vi "1.3.5-Confirm.vi"(10 "LIDAR raw data":u8) -> (0 "last measured value":u16, 1 "parser state":T1(ring), 2 "new value?":bool, 4 "angle":u8)   [LabVIEW 2010]
doc: "Finite Autonoma for parsing Lidar Raw Data"
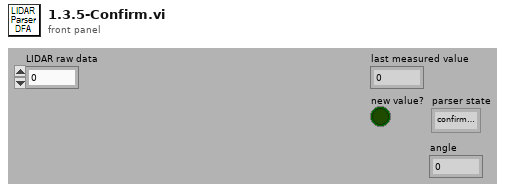
[diagram p1: front panel]
types:
  T1 = enum16{"confirm check sum", "check status byte", "read measured values", "confirm measurement", "confirm command", "read message length", "read address", "wait for \"02\""}
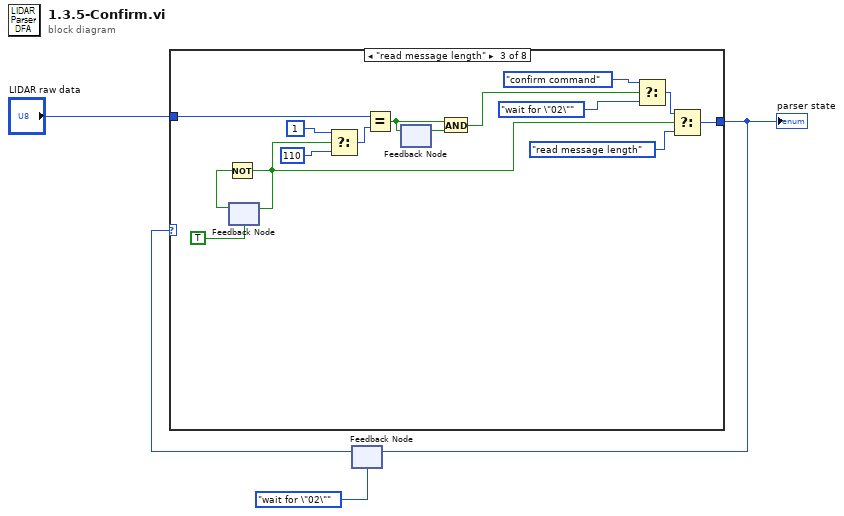
[diagram p0: block diagram]
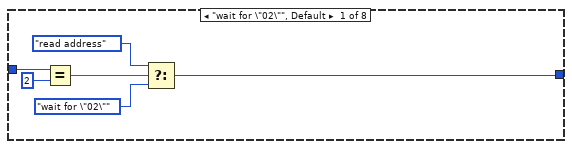
[diagram p2: hidden frame]
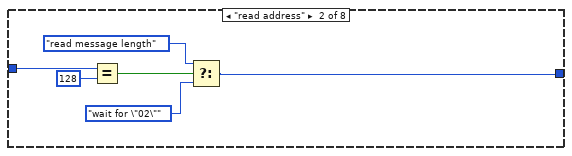
[diagram p3: hidden frame]
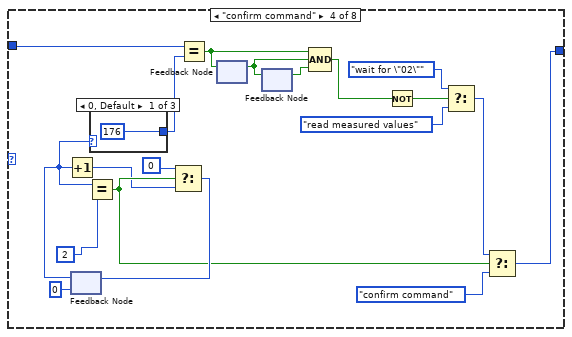
[diagram p4: hidden frame]
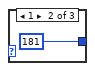
[diagram p5: hidden frame]
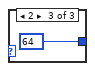
[diagram p6: hidden frame]
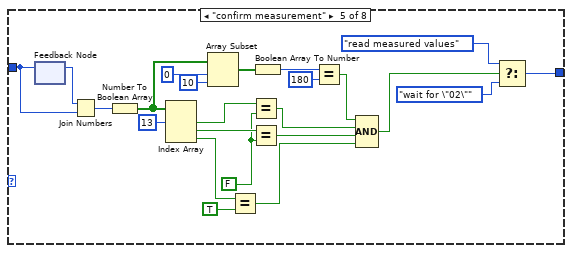
[diagram p7: hidden frame]
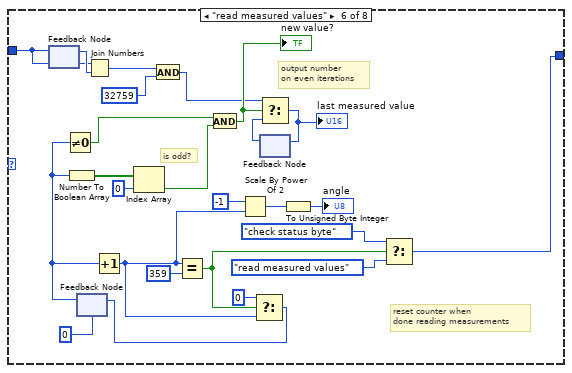
[diagram p8: hidden frame]
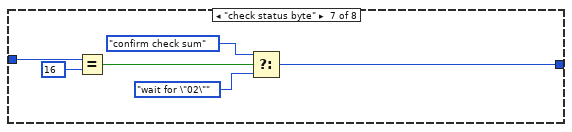
[diagram p9: hidden frame]
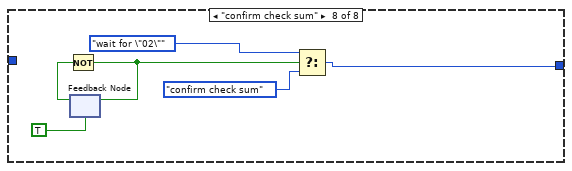
[diagram p10: hidden frame]
diagram:
  n1 = feedback #1(T1."wait for \"02\"") -> (w3:T1)
  n2 = case shown="\"read message length\"" w3 {
    tunnel: "LIDAR raw data" -> [w10 w16 w27 w50 w75 w100 w107 _]
    tunnel: [w5 w11 w29 w34 w57 w85 w102 w108] -> w2
    frame "wait for \"02\"", Default {
      n3 = Equal?(x=w10, y=i8 2) -> (x = y?=w8:bool)
      n4 = Select(t=T1."read address", s=w8, f=T1."wait for \"02\"") -> (s? t:f=w5:T1)
    }
    frame "read address" {
      n5 = Equal?(x=w16, y=u8 128) -> (x = y?=w14:bool)
      n6 = Select(t=T1."read message length", s=w14, f=T1."wait for \"02\"") -> (s? t:f=w11:T1)
    }
    frame "read message length" {
      n7 = feedback #2(TRUE) -> (w31:bool)
      n8 = Not(x=w31) -> (.not. x?=w26:bool)
      n9 = feedback-in #2(w26) -> ()
      n10 = Select(t=u8 1 ("LIDAR raw data"), s=w26, f=u8 110 ("LIDAR raw data")) -> (s? t:f=w23:u8)
      n11 = Equal?(x=w27, y=w23) -> (x = y?=w18:bool)
      n12 = feedback-in #3(w18) -> ()
      n13 = feedback #3() -> (w19:bool)  [unwired: 1 in]
      n14 = And(x=w18, y=w19) -> (x .and. y?=w21:bool)
      n15 = Select(t=T1."confirm command", s=w21, f=T1."wait for \"02\"") -> (s? t:f=w17:T1)
      n16 = Select(t=w17, s=w26, f=T1."read message length") -> (s? t:f=w29:T1)
    }
    frame "confirm command" {
      n17 = feedback #4(u8 0 ("y")) -> (w37:u8)
      n18 = Increment(x=w37) -> (x+1=w32:u8)
      n19 = Equal?(x=w37, y=u8 2) -> (x = y?=w38:bool)
      n20 = case shown="0, Default" w37 {
        tunnel: [u8 176 ("y") u8 181 ("y") u8 64 ("y")] -> w45
        frame 0, Default {
        }
        frame 1 {
        }
        frame 2 {
        }
      }
      n21 = Select(t=u8 0 ("y"), s=w38, f=w32) -> (s? t:f=w47:u8)
      n22 = feedback-in #4(w47) -> ()
      n23 = Equal?(x=w50, y=w45) -> (x = y?=w44:bool)
      n24 = feedback-in #5(w44) -> ()
      n25 = feedback #5() -> (w43:bool)  [unwired: 1 in]
      n26 = feedback-in #6(w43) -> ()
      n27 = feedback #6() -> (w42:bool)  [unwired: 1 in]
      n28 = Compound Arithmetic op=AND(w44, w43, w42) -> (w41:bool)
      n29 = Not(x=w41) -> (.not. x?=w40:bool)
      n30 = Select(t=T1."wait for \"02\"", s=w40, f=T1."read measured values") -> (s? t:f=w35:T1)
      n31 = Select(t=w35, s=w38, f=T1."confirm command") -> (s? t:f=w34:T1)
    }
    frame "confirm measurement" {
      w69 = FALSE ("y")
      n32 = feedback-in #7(w75) -> ()
      n33 = feedback #7() -> (w76:u8)  [unwired: 1 in]
      n34 = Join Numbers(hi=w76, lo=w75) -> ((hi.lo)=w74:u16)
      n35 = Number To Boolean Array(number=w74) -> (Boolean array=w64:bool[])
      n36 = Index Array(array=w64, index #1=13 ("index")) -> (element #1=w68:bool, element #2=w70:bool, element #3=w72:bool)  [unwired: 2 in]
      n37 = Array Subset(array=w64, index=0, length=10) -> (w61:bool[])
      n38 = Equal?(x=w72, y=TRUE) -> (x = y?=w65:bool)
      n39 = Equal?(x=w68, y=w69) -> (x = y?=w67:bool)
      n40 = Equal?(x=w70, y=w69) -> (x = y?=w66:bool)
      n41 = Boolean Array To Number(Boolean array=w61) -> (number=w60:u16)
      n42 = Equal?(x=w60, y=u16 180) -> (x = y?=w58:bool)
      n43 = Compound Arithmetic op=AND(w58, w67, w66, w65) -> (w56:bool)
      n44 = Select(t=T1."read measured values", s=w56, f=T1."wait for \"02\"") -> (s? t:f=w57:T1)
    }
    frame "read measured values" {
      # "is odd?"
      # "output number\non even iterations"
      # "reset counter when\ndone reading measurements"
      n45 = feedback-in #8(w100) -> ()
      n46 = feedback #8() -> (w101:u8)  [unwired: 1 in]
      n47 = feedback #9(i16 0) -> (w93:i16)
      n48 = Not Equal To 0?(x=w93) -> (x != 0?=w92:bool)
      n49 = Number To Boolean Array(number=w93) -> (Boolean array=w97:bool[])
      n50 = Join Numbers(hi=w100, lo=w101) -> ((hi.lo)=w82:u16)
      n51 = Increment(x=w93) -> (x+1=w80:i16)
      n52 = Index Array(array=w97, index=0) -> (element=w84:bool)
      n53 = And(x=w82, y=u16 32759) -> (x .and. y?=w81:u16)
      n54 = Equal?(x=w80, y=i16 359) -> (x = y?=w88:bool)
      n55 = And(x=w92, y=w84) -> (x .and. y?=w91:bool)
      "new value?" <- w91
      n56 = Scale By Power Of 2(n=-1, x=w80) -> (x*2^n=w78:i16)
      n57 = Select(t=i16 0, s=w88, f=w80) -> (s? t:f=w90:i16)
      n58 = feedback-in #9(w90) -> ()
      n59 = feedback #10() -> (w94:u16)  [unwired: 1 in]
      n60 = Select(t=w81, s=w91, f=w94) -> (s? t:f=w95:u16)
      "last measured value" <- w95
      n61 = feedback-in #10(w95) -> ()
      n62 = To Unsigned Byte Integer(number=w78) -> (unsigned 8bit integer=→"angle":u8)
      n63 = Select(t=T1."check status byte", s=w88, f=T1."read measured values") -> (s? t:f=w85:T1)
    }
    frame "check status byte" {
      n64 = Equal?(x=w107, y=u8 16) -> (x = y?=w105:bool)
      n65 = Select(t=T1."confirm check sum", s=w105, f=T1."wait for \"02\"") -> (s? t:f=w102:T1)
    }
    frame "confirm check sum" {
      n66 = feedback #11(TRUE) -> (w113:bool)
      n67 = Not(x=w113) -> (.not. x?=w111:bool)
      n68 = feedback-in #11(w111) -> ()
      n69 = Select(t=T1."wait for \"02\"", s=w111, f=T1."confirm check sum") -> (s? t:f=w108:T1)
    }
  }
  "parser state" <- w2
  n70 = feedback-in #1(w2) -> ()
